vi "ztscopeM Capture Complete Query.vi"(8 "error in":errorcluster, 11 "Instrument Handle In":i32) -> (0 "error out":errorcluster, 2 "State":i32, 3 "Instrument Handle Out":i32)   [LabVIEW 2013]
doc: "Query whether the instrument is currently capturing."
uses:
  ztscopeM.dll
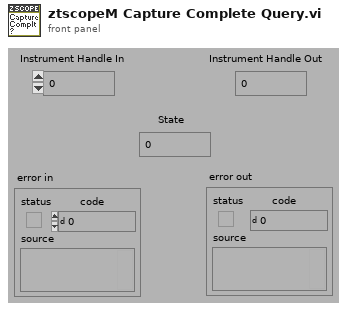
[diagram p1: front panel]
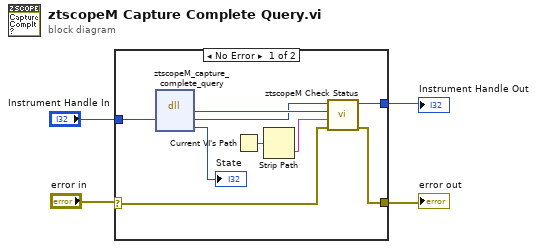
[diagram p0: block diagram]
diagram:
  n1 = case shown="No Error" "error in" {
    selector: "error in" -> [w7 w15]
    tunnel: [w5 w15] -> w1
    tunnel: "Instrument Handle In" -> [w13 w14]
    tunnel: [w6 w14] -> w3
    frame No Error {
      n2 = dll-call lib="C:/Program Files/National Instruments/instr.lib/ztscopem/ztscopeM.dll" fn="ztscopeM_capture_complete_query"("instrumentHandle"=w13) -> (w9:i32, "instrumentHandle"=w8:i32, "state"=→"State":i32)  [unwired: 4 in, 2 out]
      n3 = Current VI's Path() -> (path=w11:path)
      n4 = Strip Path(path=w11) -> (name=w10:string)  [unwired: 1 out]
      n5 = call "ztscopeM Check Status.vi"("error in"=w7, "name of VI"=w10, "status"=w9, "instrument handle in"=w8) -> ("error out"=w5:errorcluster, "instrument handle out"=w6:i32)  [unwired: 2 in]
    }
    frame Error {
    }
  }
  "Instrument Handle Out" <- w3
  "error out" <- w1
